vi "test_main_status.vi"() -> ()   [LabVIEW 2019]
uses:
  RT/RT Controls/Main Box Control.ctl
  RT/RT Controls/Top Dome Control.ctl
  RT/RT Controls/Main Box Config.ctl
  RT/RT Controls/TopBox Config.ctl
  RT/RT Controls/Main Box Status.ctl
  RT/RT Controls/Rotation Status.ctl
  RT/RT Controls/Last Rotation.ctl
  RT/RT Controls/Homing State.ctl
  RT/RT Controls/Top Dome Status.ctl
panel:
  in  "TopDomeStat":T1 {"LowerDoorEl" format="%.2f"; "UpperDoorEl" format="%.2f"}
  in  "MainBoxStatus":T2 {"LastAZ" format="%.2f"; "CurAZ" format="%.2f"}
  in  "TopConf":T6={"WatchdogTim"=600, "RainEn"=FALSE, "DoorMoveTO"=10, "AutoShutEn"=FALSE, "DirRevDel"=5, "UpperClosedEnc"=0, "UpperOpenEnc"=0, "LowerClosedEnc"=0, "LowerOpenEnc"=0, "RainTim"=60, "DropoutTim"=5}
  in  "MainBoxConfig":T7={"WatchdogTim"=600, "DirRevDel"=5, "Coast"=0.0, "HSThres"=0.0, "EncCounts360"=0, "HomePos"=0.0, "EncRefDeg"=0.0, "EncRefCounts"=0, "Tol"=0.0, "CloudEn"=FALSE, "AutoShutEn"=FALSE, "RainTim"=5, "AZTimeout"=300, "AZEncPol"=enum."Positive"} {"Tol" format="%.2f"; "EncRefDeg" format="%.2f"; "HomePos" format="%.2f"; "HSThres" format="%.2f"; "Coast" format="%.2f"}
  in  "TopDomeCtrl":T8
  in  "MainBoxCtrl":T9
  out "FullStat":string
  out "ShortStat":string
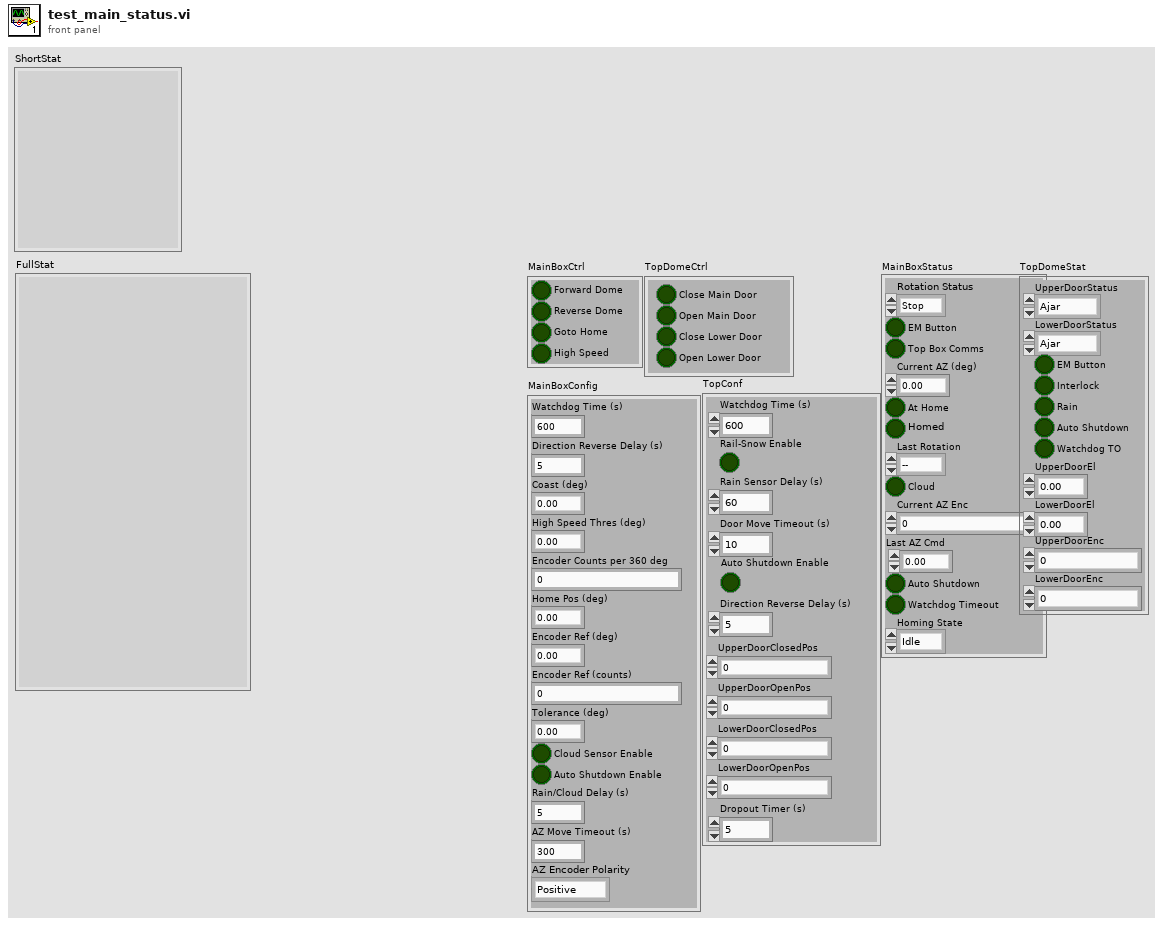
[diagram p1: front panel]
types:
  T1 = typedef "Top Dome Status.ctl" = cluster{"UpperDoorStatus":enum16{"Ajar", "Open", "Shut", "Error"}, "LowerDoorStatus":enum16{"Ajar", "Shut", "Open", "Error"}, "EM Button":bool, "WDTime":bool, "AutoShut":bool, "Rain":bool, "Interlock":bool, "UpperDoorEl":dbl, "LowerDoorEl":dbl, "UpperDoorEnc":u64, "LowerDoorEnc":u64}
  T2 = typedef "Main Box Status.ctl" = cluster{"RotStatus":T3, "EMButton":bool, "TopComms":bool, "CurAZ":dbl, "At Home":bool, "Homed":bool, "LastRot":T4, "Cloud":bool, "CurAZEnc":u64, "LastAZ":dbl, "AutoShut":bool, "WDTime":bool, "HomeState":T5}
  T3 = typedef "Rotation Status.ctl" = enum16{"Stop", "Left", "Right", "Homing"}
  T4 = typedef "Last Rotation.ctl" = enum16{"--", "RR", "RL"}
  T5 = typedef "Homing State.ctl" = enum16{"Idle", "SlewFwd", "SlewRev", "SeekFwd", "SeekRev", "AtHome", "FwdWait", "RevWait"}
  T6 = typedef "TopBox Config.ctl" = cluster{"WatchdogTim":i32, "RainEn":bool, "DoorMoveTO":i32, "AutoShutEn":bool, "DirRevDel":i32, "UpperClosedEnc":u64, "UpperOpenEnc":u64, "LowerClosedEnc":u64, "LowerOpenEnc":u64, "RainTim":i32, "DropoutTim":i32}
  T7 = typedef "Main Box Config.ctl" = cluster{"WatchdogTim":i32, "DirRevDel":i32, "Coast":dbl, "HSThres":dbl, "EncCounts360":u64, "HomePos":dbl, "EncRefDeg":dbl, "EncRefCounts":u64, "Tol":dbl, "CloudEn":bool, "AutoShutEn":bool, "RainTim":i32, "AZTimeout":i32, "AZEncPol":enum16{"Positive", "Negative"}}
  T8 = typedef "Top Dome Control.ctl" = cluster{"OpenLowerDoor":bool, "CloseLowerDoor":bool, "OpenMainDoor":bool, "CloseMainDoor":bool}
  T9 = typedef "Main Box Control.ctl" = cluster{"ForwardDome":bool, "ReverseDome":bool, "GotoHome":bool, "HighSpeed":bool}
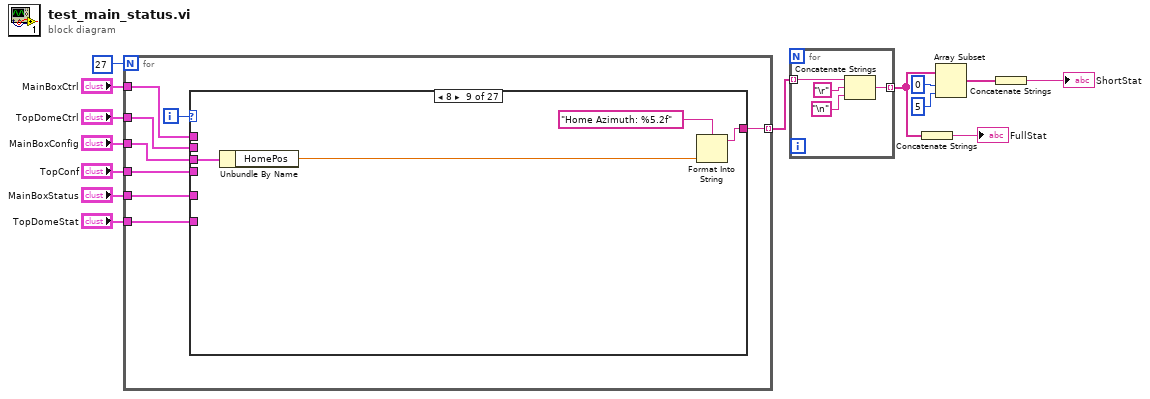
[diagram p0: block diagram]
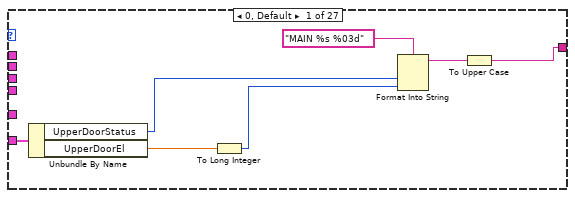
[diagram p2: hidden frame]
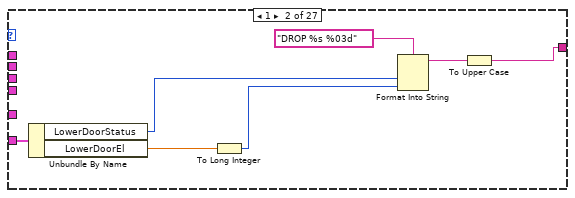
[diagram p3: hidden frame]
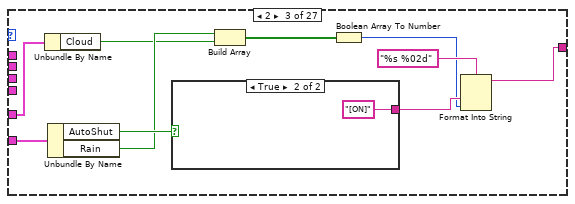
[diagram p4: hidden frame]
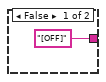
[diagram p5: hidden frame]
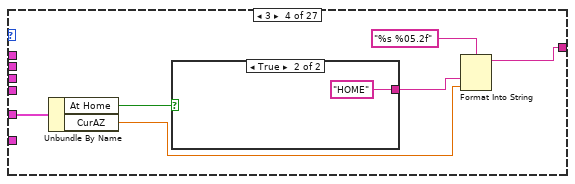
[diagram p6: hidden frame]
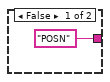
[diagram p7: hidden frame]
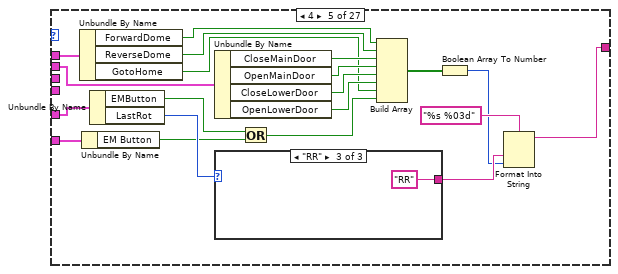
[diagram p8: hidden frame]
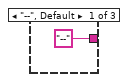
[diagram p9: hidden frame]
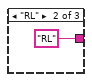
[diagram p10: hidden frame]
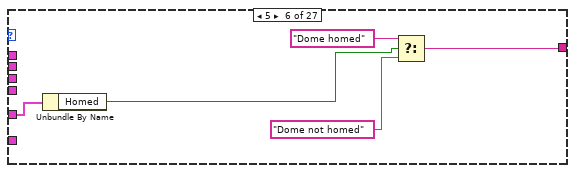
[diagram p11: hidden frame]
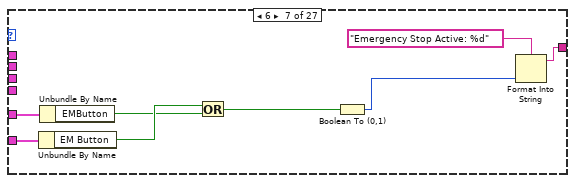
[diagram p12: hidden frame]
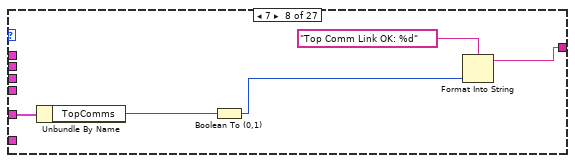
[diagram p13: hidden frame]
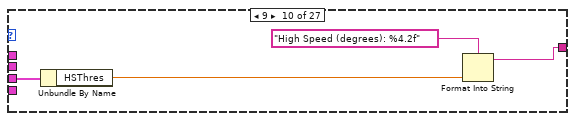
[diagram p14: hidden frame]
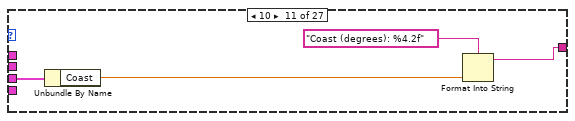
[diagram p15: hidden frame]
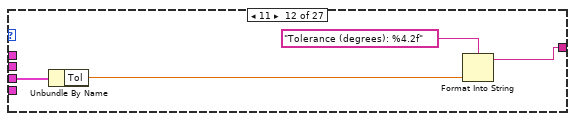
[diagram p16: hidden frame]
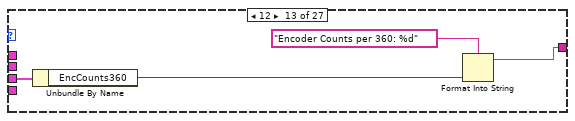
[diagram p17: hidden frame]
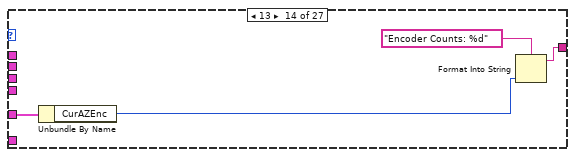
[diagram p18: hidden frame]
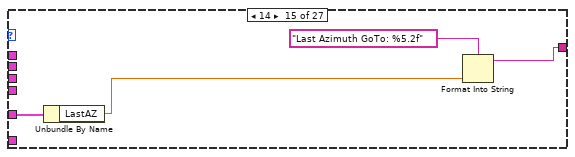
[diagram p19: hidden frame]
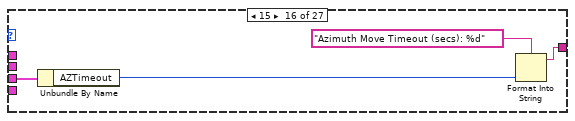
[diagram p20: hidden frame]
diagram:
  n1 = for {
    N: 27 -> [_]
    tunnel: "TopDomeStat" -> [w22]
    tunnel: [w20] -> w10 mode=indexing
    tunnel: "MainBoxStatus" -> [w19]
    tunnel: "MainBoxCtrl" -> [w18]
    tunnel: "TopDomeCtrl" -> [w17]
    tunnel: "MainBoxConfig" -> [w16]
    tunnel: "TopConf" -> [w15]
    i -> [w21]
    n2 = case shown="8" w21 {
      tunnel: w22 -> [w29 w36 w46 _ w62 _ w89 _ _ _ _ _ _ _ _ _ w132 _ _ _ _ _ _ _ _ _ _]
      tunnel: [w26 w33 w41 w49 w59 w81 w91 w96 w100 w104 w108 w112 w116 w120 w124 w128 w133 w138 w142 w146 w150 w154 w158 w162 w166 w170 w172] -> w20
      tunnel: w19 -> [_ _ w43 w54 w76 w84 w90 w95 _ _ _ _ _ w118 w122 _ _ _ _ _ _ _ _ _ _ _ w178]
      tunnel: w18 -> [_ _ _ _ w65 _ _ _ _ _ _ _ _ _ _ _ _ _ _ _ _ _ _ _ _ _ _]
      tunnel: w17 -> [_ _ _ _ w64 _ _ _ _ _ _ _ _ _ _ _ _ _ _ _ _ _ _ _ _ _ _]
      tunnel: w16 -> [_ _ _ _ _ _ _ _ w99 w103 w107 w111 w115 _ _ w126 _ w135 _ _ _ _ _ _ _ _ _]
      tunnel: w15 -> [_ _ _ _ _ _ _ _ _ _ _ _ _ _ _ _ _ _ w141 w145 w149 w153 w157 w161 w165 w169 _]
      frame 0, Default {
        n3 = Unbundle By Name(w29) -> ("UpperDoorStatus"=w25:enum16{"Ajar", "Open", "Shut", "Error"}, "UpperDoorEl"=w24:dbl)
        n4 = To Long Integer(number=w24) -> (32bit integer=w23:i32)
        n5 = Format Into String(format string="MAIN %s %03d", w25, w23) -> (resulting string=w27:string)  [unwired: 2 in, 1 out]
        n6 = To Upper Case(1:w27) -> (0:w26:string)
      }
      frame 1 {
        n7 = Unbundle By Name(w36) -> ("LowerDoorStatus"=w32:enum16{"Ajar", "Shut", "Open", "Error"}, "LowerDoorEl"=w31:dbl)
        n8 = To Long Integer(number=w31) -> (32bit integer=w30:i32)
        n9 = Format Into String(format string="DROP %s %03d", w32, w30) -> (resulting string=w34:string)  [unwired: 2 in, 1 out]
        n10 = To Upper Case(1:w34) -> (0:w33:string)
      }
      frame 2 {
        n11 = Unbundle By Name(w43) -> ("Cloud"=w38:bool)
        n12 = Unbundle By Name(w46) -> ("AutoShut"=w45:bool, "Rain"=w39:bool)
        n13 = case shown="True" w45 {
          tunnel: ["[OFF]" ("string") "[ON]" ("string")] -> w42
          frame False {
          }
          frame True {
          }
        }
        n14 = Build Array(w39, w38) -> (w40:bool[])
        n15 = Boolean Array To Number(Boolean array=w40) -> (number=w37:u32)
        n16 = Format Into String(format string="%s %02d", w42, w37) -> (resulting string=w41:string)  [unwired: 2 in, 1 out]
      }
      frame 3 {
        n17 = Unbundle By Name(w54) -> ("At Home"=w53:bool, "CurAZ"=w50:dbl)
        n18 = case shown="True" w53 {
          tunnel: ["POSN" ("string") "HOME" ("string")] -> w52
          frame False {
          }
          frame True {
          }
        }
        n19 = Format Into String(format string="%s %05.2f", w52, w50) -> (resulting string=w49:string)  [unwired: 2 in, 1 out]
      }
      frame 4 {
        n20 = Unbundle By Name(w65) -> ("ForwardDome"=w72:bool, "ReverseDome"=w71:bool, "GotoHome"=w66:bool)
        n21 = Unbundle By Name(w62) -> ("EM Button"=w58:bool)
        n22 = Unbundle By Name(w76) -> ("EMButton"=w57:bool, "LastRot"=w75:T4)
        n23 = Unbundle By Name(w64) -> ("CloseMainDoor"=w70:bool, "OpenMainDoor"=w69:bool, "CloseLowerDoor"=w68:bool, "OpenLowerDoor"=w67:bool)
        n24 = case shown="\"RR\"" w75 {
          tunnel: ["--" ("string") "RL" ("string") "RR" ("string")] -> w73
          frame "--", Default {
          }
          frame "RL" {
          }
          frame "RR" {
          }
        }
        n25 = Or(x=w57, y=w58) -> (x .or. y?=w63:bool)
        n26 = Build Array(w72, w71, w70, w69, w68, w67, w66, w63) -> (w61:bool[])
        n27 = Boolean Array To Number(Boolean array=w61) -> (number=w60:u32)
        n28 = Format Into String(format string="%s %03d", w73, w60) -> (resulting string=w59:string)  [unwired: 2 in, 1 out]
      }
      frame 5 {
        n29 = Unbundle By Name(w84) -> ("Homed"=w83:bool)
        n30 = Select(t="Dome homed", s=w83, f="Dome not homed") -> (s? t:f=w81:string)
      }
      frame 6 {
        n31 = Unbundle By Name(w89) -> ("EM Button"=w88:bool)
        n32 = Unbundle By Name(w90) -> ("EMButton"=w87:bool)
        n33 = Or(x=w88, y=w87) -> (x .or. y?=w86:bool)
        n34 = Boolean To (0,1)(Boolean=w86) -> (0, 1=w85:i16)
        n35 = Format Into String(format string="Emergency Stop Active: %d", w85) -> (resulting string=w91:string)  [unwired: 2 in, 1 out]
      }
      frame 7 {
        n36 = Unbundle By Name(w95) -> ("TopComms"=w93:bool)
        n37 = Boolean To (0,1)(Boolean=w93) -> (0, 1=w94:i16)
        n38 = Format Into String(format string="Top Comm Link OK: %d", w94) -> (resulting string=w96:string)  [unwired: 2 in, 1 out]
      }
      frame 8 {
        n39 = Unbundle By Name(w99) -> ("HomePos"=w98:dbl)
        n40 = Format Into String(format string="Home Azimuth: %5.2f", w98) -> (resulting string=w100:string)  [unwired: 2 in, 1 out]
      }
      frame 9 {
        n41 = Unbundle By Name(w103) -> ("HSThres"=w102:dbl)
        n42 = Format Into String(format string="High Speed (degrees): %4.2f", w102) -> (resulting string=w104:string)  [unwired: 2 in, 1 out]
      }
      frame 10 {
        n43 = Unbundle By Name(w107) -> ("Coast"=w106:dbl)
        n44 = Format Into String(format string="Coast (degrees): %4.2f", w106) -> (resulting string=w108:string)  [unwired: 2 in, 1 out]
      }
      frame 11 {
        n45 = Unbundle By Name(w111) -> ("Tol"=w110:dbl)
        n46 = Format Into String(format string="Tolerance (degrees): %4.2f", w110) -> (resulting string=w112:string)  [unwired: 2 in, 1 out]
      }
      frame 12 {
        n47 = Unbundle By Name(w115) -> ("EncCounts360"=w114:u64)
        n48 = Format Into String(format string="Encoder Counts per 360: %d", w114) -> (resulting string=w116:string)  [unwired: 2 in, 1 out]
      }
      frame 13 {
        n49 = Unbundle By Name(w118) -> ("CurAZEnc"=w119:u64)
        n50 = Format Into String(format string="Encoder Counts: %d", w119) -> (resulting string=w120:string)  [unwired: 2 in, 1 out]
      }
      frame 14 {
        n51 = Unbundle By Name(w122) -> ("LastAZ"=w123:dbl)
        n52 = Format Into String(format string="Last Azimuth GoTo: %5.2f", w123) -> (resulting string=w124:string)  [unwired: 2 in, 1 out]
      }
      frame 15 {
        n53 = Unbundle By Name(w126) -> ("AZTimeout"=w127:i32)
        n54 = Format Into String(format string="Azimuth Move Timeout (secs): %d", w127) -> (resulting string=w128:string)  [unwired: 2 in, 1 out]
      }
      frame 16 {
        n55 = Unbundle By Name(w132) -> ("Rain"=w131:bool)
        n56 = Boolean To (0,1)(Boolean=w131) -> (0, 1=w130:i16)
        n57 = Format Into String(format string="Rain-Snow enabled: %d", w130) -> (resulting string=w133:string)  [unwired: 2 in, 1 out]
      }
      frame 17 {
        n58 = Unbundle By Name(w135) -> ("CloudEn"=w137:bool)
        n59 = Boolean To (0,1)(Boolean=w137) -> (0, 1=w136:i16)
        n60 = Format Into String(format string="Cloud Sensor enabled: %d", w136) -> (resulting string=w138:string)  [unwired: 2 in, 1 out]
      }
      frame 18 {
        n61 = Unbundle By Name(w141) -> ("WatchdogTim"=w140:i32)
        n62 = Format Into String(format string="Watchdog Reset Time: %d", w140) -> (resulting string=w142:string)  [unwired: 2 in, 1 out]
      }
      frame 19 {
        n63 = Unbundle By Name(w145) -> ("DropoutTim"=w144:i32)
        n64 = Format Into String(format string="Dropout Timer: %d", w144) -> (resulting string=w146:string)  [unwired: 2 in, 1 out]
      }
      frame 20 {
        n65 = Unbundle By Name(w149) -> ("DirRevDel"=w148:i32)
        n66 = Format Into String(format string="Reverse Delay: %d", w148) -> (resulting string=w150:string)  [unwired: 2 in, 1 out]
      }
      frame 21 {
        n67 = Unbundle By Name(w153) -> ("UpperClosedEnc"=w152:u64)
        n68 = Format Into String(format string="Main Door Encoder Closed: %d", w152) -> (resulting string=w154:string)  [unwired: 2 in, 1 out]
      }
      frame 22 {
        n69 = Unbundle By Name(w157) -> ("UpperOpenEnc"=w156:u64)
        n70 = Format Into String(format string="Main Door Encoder Opened: %d", w156) -> (resulting string=w158:string)  [unwired: 2 in, 1 out]
      }
      frame 23 {
        n71 = Unbundle By Name(w161) -> ("LowerClosedEnc"=w160:u64)
        n72 = Format Into String(format string="Dropout Encoder Closed: %d", w160) -> (resulting string=w162:string)  [unwired: 2 in, 1 out]
      }
      frame 24 {
        n73 = Unbundle By Name(w165) -> ("LowerOpenEnc"=w164:u64)
        n74 = Format Into String(format string="Dropout Encoder Opened: %d", w164) -> (resulting string=w166:string)  [unwired: 2 in, 1 out]
      }
      frame 25 {
        n75 = Unbundle By Name(w169) -> ("DoorMoveTO"=w168:i32)
        n76 = Format Into String(format string="Door Move Timeout (secs): %d", w168) -> (resulting string=w170:string)  [unwired: 2 in, 1 out]
      }
      frame 26 {
        n77 = Unbundle By Name(w178) -> ("Homed"=w177:bool)
        n78 = Select(t="True", s=w177, f="False") -> (s? t:f=w173:string)
        n79 = Format Into String(format string="Dome has been homed: %s", w173) -> (resulting string=w172:string)  [unwired: 2 in, 1 out]
      }
    }
  }
  n80 = for {
    tunnel: w10 -> [w182] mode=indexing
    tunnel: [w179] -> w8 mode=indexing
    n81 = Concatenate Strings(w182, "\r", "\n") -> (w179:string)
  }
  n82 = Concatenate Strings(w8) -> (→"FullStat":string)
  n83 = Array Subset(array=w8, index=0, length=5) -> (w7:string[])
  n84 = Concatenate Strings(w7) -> (→"ShortStat":string)
